vi "initialize.vi"(8 "error in (no error)":errorcluster, 11 "HelioUpdateMH100803 in":refnum<class "HelioUpdateMH100803.lvclass">) -> (0 "error out":errorcluster, 3 "HelioUpdateMH100803 out":refnum<class "HelioUpdateMH100803.lvclass">)   [LabVIEW 2010, in "HelioUpdateMH100803.lvclass"]
uses:
  HelioUpdateMH100803.lvclass
  HelioUpdateMH100803.lvclass/HelioUpdateMH100803.ctl
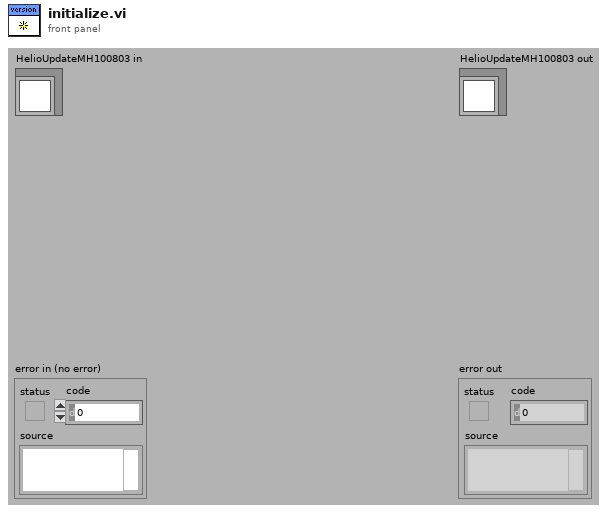
[diagram p1: front panel]
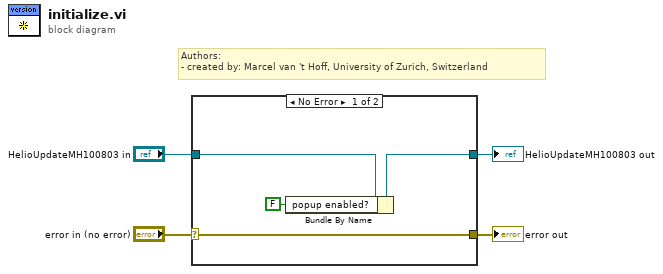
[diagram p0: block diagram]
diagram:
  # "Authors: \n- created by: Marcel van 't Hoff, University of Zurich, Switzerland"
  n1 = case shown="No Error" "error in (no error)" {
    selector: "error in (no error)" -> [w8 w10]
    tunnel: [w8 w10] -> w3
    tunnel: [w6 w9] -> w1
    tunnel: "HelioUpdateMH100803 in" -> [w7 w9]
    frame No Error {
      n2 = Bundle By Name(cluster=w7, "popup enabled?"=FALSE) -> (w6:refnum<class "HelioUpdateMH100803.lvclass">)
    }
    frame Error {
    }
  }
  "error out" <- w3
  "HelioUpdateMH100803 out" <- w1
